vi "UIRef.vi"(8 "error in":errorcluster, 11 "Submodule EOL":refnum<class "Submodule EOL.lvclass">) -> (0 "error out":errorcluster, 2 "VI refnum":refnum<vi>, 3 "Submodule EOL out":refnum<class "Submodule EOL.lvclass">)   [LabVIEW 2025, in "Submodule EOL.lvlib" / "Submodule EOL.lvclass"]
doc: "Stores the static reference to the UI of the node.Copyright 2017 National Instruments Corporation\n\nLicensed under the Apache License, Version 2.0 (the \"License\"); you may not use this file except in compliance with the License. You may obtain a copy of the License at http://www.apache.org/licenses/LICENSE-2.0\nUnless required by applicable law or agreed to in writing, software distributed under the License is distributed on an \"AS IS\" BASIS, WITHOUT WARRANTIES OR CONDITIONS OF ANY KIND, either express or implied. See the License for the specific language governing permissions and limitations under the License."
uses:
  Submodule EOL.lvclass
  Submodule EOL UI.vi
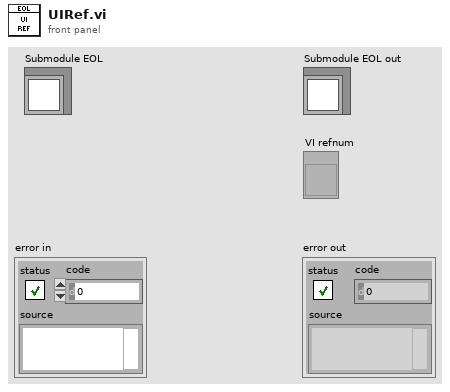
[diagram p1: front panel]
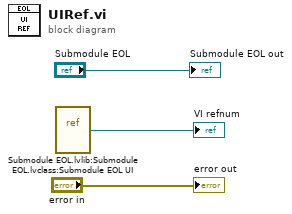
[diagram p0: block diagram]
diagram:
  n1 = vi-ref "Submodule EOL.lvlib:Submodule EOL.lvclass:Submodule EOL UI.vi"() -> (→"VI refnum":refnum<vi>)
  "error out" <- "error in"
  "Submodule EOL out" <- "Submodule EOL"
